vi "WLAN - niVST - RFSA - Measure.vi"(0 "IVI Refnum in":refnum<k15>="RIO0", 1 "Channel Bandwidth(Hz)":dbl=20000000.0, 2 "Path Loss dB":dbl=0.1, 3 "#Avg":i32=1, 6 "Power Level(dBm)":dbl=-10.0, 7 "Spectrum Meas Ref":T9, 8 "NIStandard":T1=enum."80211B/G(DSSS)", 10 "Center Frequency(Hz)":dbl=5190000000.0, 11 "IQ Measurement Ref":T9) -> (13 "Mod Result":T2={"EVM"=-53.23630011850784, "RMS POWER"=-20.854257366141734, "FREQ ERR PPm"=0.0031004693085368165, "Clock ERR PPm"=1.9815491854025864}, 14 "IVI Refnum out":refnum<k15>="RIO0", 15 "SMM":dbl, 16 "Margin VECTOR":dbl[](array[numeric]), 17 "Spectrum Meas Ref out":T9, 18 "IQ Measurement Ref out":T9, 19 "error out":errorcluster={"status"=TRUE, "code"=-42926, "source"="Property Node (arg 10) in niWLAN - OPPO - 80211abgnIQMeasurementsSettings.vi->WLAN - niVST - RFSA - Measure.vi->WLAN - OPPO - UUT(Tx).vi"})   [LabVIEW 2012]
uses:
  <vilib>/RF Toolkits/WLAN/analysis/controls/wlanv1 Analysis Refnum.ctl
  TV/RW/Includes/WLAN - TV - OPPO - RW - INC - TV_IQComposite_11N.ctl
  TV/RW/Includes/WLAN - TV - RW - INC - TV_OFDM Demod.ctl
  TV/RW/Includes/WLAN - TV - OPPO - RW - INC - TV_IQComposite_11B.ctl
  TV/RW/Includes/WLAN - TV - RW - INC - TV_DSSS Demod.ctl
  TV/RW/Includes/WLAN - TV - OPPO - RW - INC - TV_IQComposite_11A.ctl
  TV/RW/Includes/WLAN - TV - OPPO - RW - INC - TV_IQComposite_11AC.ctl
  TV/RW/Includes/WLAN - TV - RW - INC - Tx_IQModResult.ctl
  TV/RW/Includes/WLAN - NIStandardDefine.ctl
panel:
  in  "TV_IQComposite_11AC":T3={"Standard"=4, "OFDM Advanced Controls"={"OFDM Auto Compute Acquisition Length Enabled"=1, "OFDM Maximum Symbols Used"=16, "OFDM Time Tracking Enabled"=0, "OFDM Channel Tracking Enabled"=0, "OFDM Amplitude Tracking Enabled"=1, "OFDM CFO Estimation Method"=1, "OFDM Phase Tracking Method"=0, "OFDM Header Detection Enabled"=1, "OFDM MAC FCS Check Enabled"=0, "#Avg"=10, "#Iterations"=10}, "Measurement Enabled"=TRUE, "#Packets"=0, "Center Frequency(Hz)"=0.0, "Guard Interval (s)"=0.0, "FEC Coding Type"=0, "Generation Parameters"={"Channel BW(Hz)"=20000000.0, "MCS Index"=0, "OFDM Payload Length (bytes)"=4024, "Idle Interval(S)"=0.0, "N_SS"=0}, "Power Level(dBm)"=0.0} {"Generation Parameters"."Channel BW(Hz)" items=["5M"=5000000.0, "10M"=10000000.0, "20M"=20000000.0, "40M"=40000000.0, "80M"=80000000.0, "160M"=160000000.0]; "FEC Coding Type" items=["BCC", "LDPC"]; "Center Frequency(Hz)" format="%#_6p"; "OFDM Advanced Controls"."OFDM Phase Tracking Method" items=["Standard", "Instantaneous", "None", "Standard with Cubic Spline Fit"]; "OFDM Advanced Controls"."OFDM CFO Estimation Method" items=["Preamble Only", "Preamble and Data"]; "OFDM Advanced Controls"."OFDM Channel Tracking Enabled" items=["False", "True"]; "OFDM Advanced Controls"."OFDM Amplitude Tracking Enabled" items=["False", "True"]; "OFDM Advanced Controls"."OFDM Time Tracking Enabled" items=["True"=1, "False"=0]; "OFDM Advanced Controls"."OFDM Auto Compute Acquisition Length Enabled" items=["False", "True"]; "OFDM Advanced Controls"."OFDM MAC FCS Check Enabled" items=["False", "True"]; "OFDM Advanced Controls"."OFDM Header Detection Enabled" items=["False", "True"]; "Standard" items=["80211A/G/J/P OFDM", "80211B/G DSSS", "80211G DSSSOFDM", "80211N MIMOOFDM", "80211AC MIMOOFDM"]}
  in  "IQComp_11AG OFDM":T5={"Standard"=0, "OFDM Advanced Controls"={"OFDM Auto Compute Acquisition Length Enabled"=0, "OFDM Maximum Symbols Used"=16, "OFDM Time Tracking Enabled"=0, "OFDM Channel Tracking Enabled"=0, "OFDM Amplitude Tracking Enabled"=1, "OFDM CFO Estimation Method"=1, "OFDM Phase Tracking Method"=0, "OFDM Header Detection Enabled"=1, "OFDM MAC FCS Check Enabled"=0, "#Avg"=0, "#Iterations"=10}, "Measurement  Enabled ?"=FALSE, "#Packets"=0, "Center Frequency(Hz)"=0.0, "Power Level(dBm)"=0.0, "Payload Control"={"OFDM Data Rate (Mbps)"=0, "OFDM Payload Length (bytes)"=0, "Idle Interval (s)"=0.0}} {"Payload Control"."OFDM Data Rate (Mbps)" items=["6", "9", "12", "18", "24", "36", "48", "54"]; "Center Frequency(Hz)" format="%#_6p"; "OFDM Advanced Controls"."OFDM Phase Tracking Method" items=["Standard", "Instantaneous", "None", "Standard with Cubic Spline Fit"]; "OFDM Advanced Controls"."OFDM CFO Estimation Method" items=["Preamble Only", "Preamble and Data"]; "OFDM Advanced Controls"."OFDM Channel Tracking Enabled" items=["False", "True"]; "OFDM Advanced Controls"."OFDM Amplitude Tracking Enabled" items=["False", "True"]; "OFDM Advanced Controls"."OFDM Time Tracking Enabled" items=["True"=1, "False"=0]; "OFDM Advanced Controls"."OFDM Auto Compute Acquisition Length Enabled" items=["False", "True"]; "OFDM Advanced Controls"."OFDM MAC FCS Check Enabled" items=["False", "True"]; "OFDM Advanced Controls"."OFDM Header Detection Enabled" items=["False", "True"]; "Standard" items=["80211A/G/J/P OFDM", "80211B/G DSSS", "80211G DSSSOFDM", "80211N MIMOOFDM", "80211AC MIMOOFDM"]}
  in  "TV_IQComposite_11B":T6={"Standard"=1, "DSSS Demod Parameters"={"DSSS Auto Compute Acquisition Length Enabled"=0, "DSSS Equalization Enabled"=0, "DSSS Header Detection Enabled"=1, "DSSS MAC FCS Check Enabled"=0, "DSSS Measurement Start Location"=0, "DSSS Phase Tracking Method"=0, "DSSS Maximum Chips Used"=1000, "DSSS Reference Pulse Shaping Filter"=3, "DSSS Reference Pulse Shaping Filter Coefficient"=0.5, "# Avg"=1024, "# Iterations"=1024, "DSSS Power Ramp Enabled"=0}, "Measurement Enabled ? "=FALSE, "Power Level(dBm)"=0.0, "Center Frequency(Hz)"=0.0, "DSSS Generate Parameters"={"DSSS Data Rate (Mbps)"=0, "DSSS Payload Length (bytes)"=1024, "Idle Interval(S)"=0.0}} {"DSSS Generate Parameters"."DSSS Data Rate (Mbps)" items=["1", "2", "5.5 CCK", "5.5 PBCC", "11 CCK", "11 PBCC", "22", "33"]; "Center Frequency(Hz)" format="%#_6p"; "DSSS Demod Parameters"."DSSS Power Ramp Enabled" items=["False", "True"]; "DSSS Demod Parameters"."DSSS Auto Compute Acquisition Length Enabled" items=["False", "True"]; "DSSS Demod Parameters"."DSSS Phase Tracking Method" items=["Standard", "Instantaneous"]; "DSSS Demod Parameters"."DSSS Equalization Enabled" items=["False", "True"]; "DSSS Demod Parameters"."DSSS Reference Pulse Shaping Filter" items=["Rectangular", "Raised Cosine", "Root Raised Cosine", "Gaussian"]; "DSSS Demod Parameters"."DSSS MAC FCS Check Enabled" items=["False", "True"]; "DSSS Demod Parameters"."DSSS Header Detection Enabled" items=["False", "True"]; "Standard" items=["80211A/G/J/P OFDM", "80211B/G DSSS", "80211G DSSSOFDM", "80211N MIMOOFDM", "80211AC MIMOOFDM"]}
  in  "TV_IQComposite_11N":T8={"Standard"=3, "OFDM Advanced Controls"={"OFDM Auto Compute Acquisition Length Enabled"=0, "OFDM Maximum Symbols Used"=0, "OFDM Time Tracking Enabled"=0, "OFDM Channel Tracking Enabled"=0, "OFDM Amplitude Tracking Enabled"=1, "OFDM CFO Estimation Method"=1, "OFDM Phase Tracking Method"=0, "OFDM Header Detection Enabled"=1, "OFDM MAC FCS Check Enabled"=0, "#Avg"=10, "#Iterations"=10}, "Measurement Enabled"=FALSE, "#Packets"=0, "Guard Interval (s)"=0.0, "FEC Coding Type"=0, "80211n PLCP Frame Format"=0, "Generation Parameters"={"Channel Bandwidth(Hz)"=20000000.0, "MCS Index"=0, "OFDM Payload Length (bytes)"=4024, "Idle Interval(S)"=0.0}, "Power Level(dBm)"=0.0, "Center Frequency(Hz)"=0.0} {"Center Frequency(Hz)" format="%#_6p"; "Generation Parameters"."Channel Bandwidth(Hz)" items=["5M"=5000000.0, "10M"=10000000.0, "20M"=20000000.0, "40M"=40000000.0, "80M"=80000000.0, "160M"=160000000.0]; "80211n PLCP Frame Format" items=["Mixed Format", "Greenfield Format"]; "FEC Coding Type" items=["BCC", "LDPC"]; "OFDM Advanced Controls"."OFDM Phase Tracking Method" items=["Standard", "Instantaneous", "None", "Standard with Cubic Spline Fit"]; "OFDM Advanced Controls"."OFDM CFO Estimation Method" items=["Preamble Only", "Preamble and Data"]; "OFDM Advanced Controls"."OFDM Channel Tracking Enabled" items=["False", "True"]; "OFDM Advanced Controls"."OFDM Amplitude Tracking Enabled" items=["False", "True"]; "OFDM Advanced Controls"."OFDM Time Tracking Enabled" items=["True"=1, "False"=0]; "OFDM Advanced Controls"."OFDM Auto Compute Acquisition Length Enabled" items=["False", "True"]; "OFDM Advanced Controls"."OFDM MAC FCS Check Enabled" items=["False", "True"]; "OFDM Advanced Controls"."OFDM Header Detection Enabled" items=["False", "True"]; "Standard" items=["80211A/G/J/P OFDM", "80211B/G DSSS", "80211G DSSSOFDM", "80211N MIMOOFDM", "80211AC MIMOOFDM"]}
  in  "Data Rate (Mbps)":i32
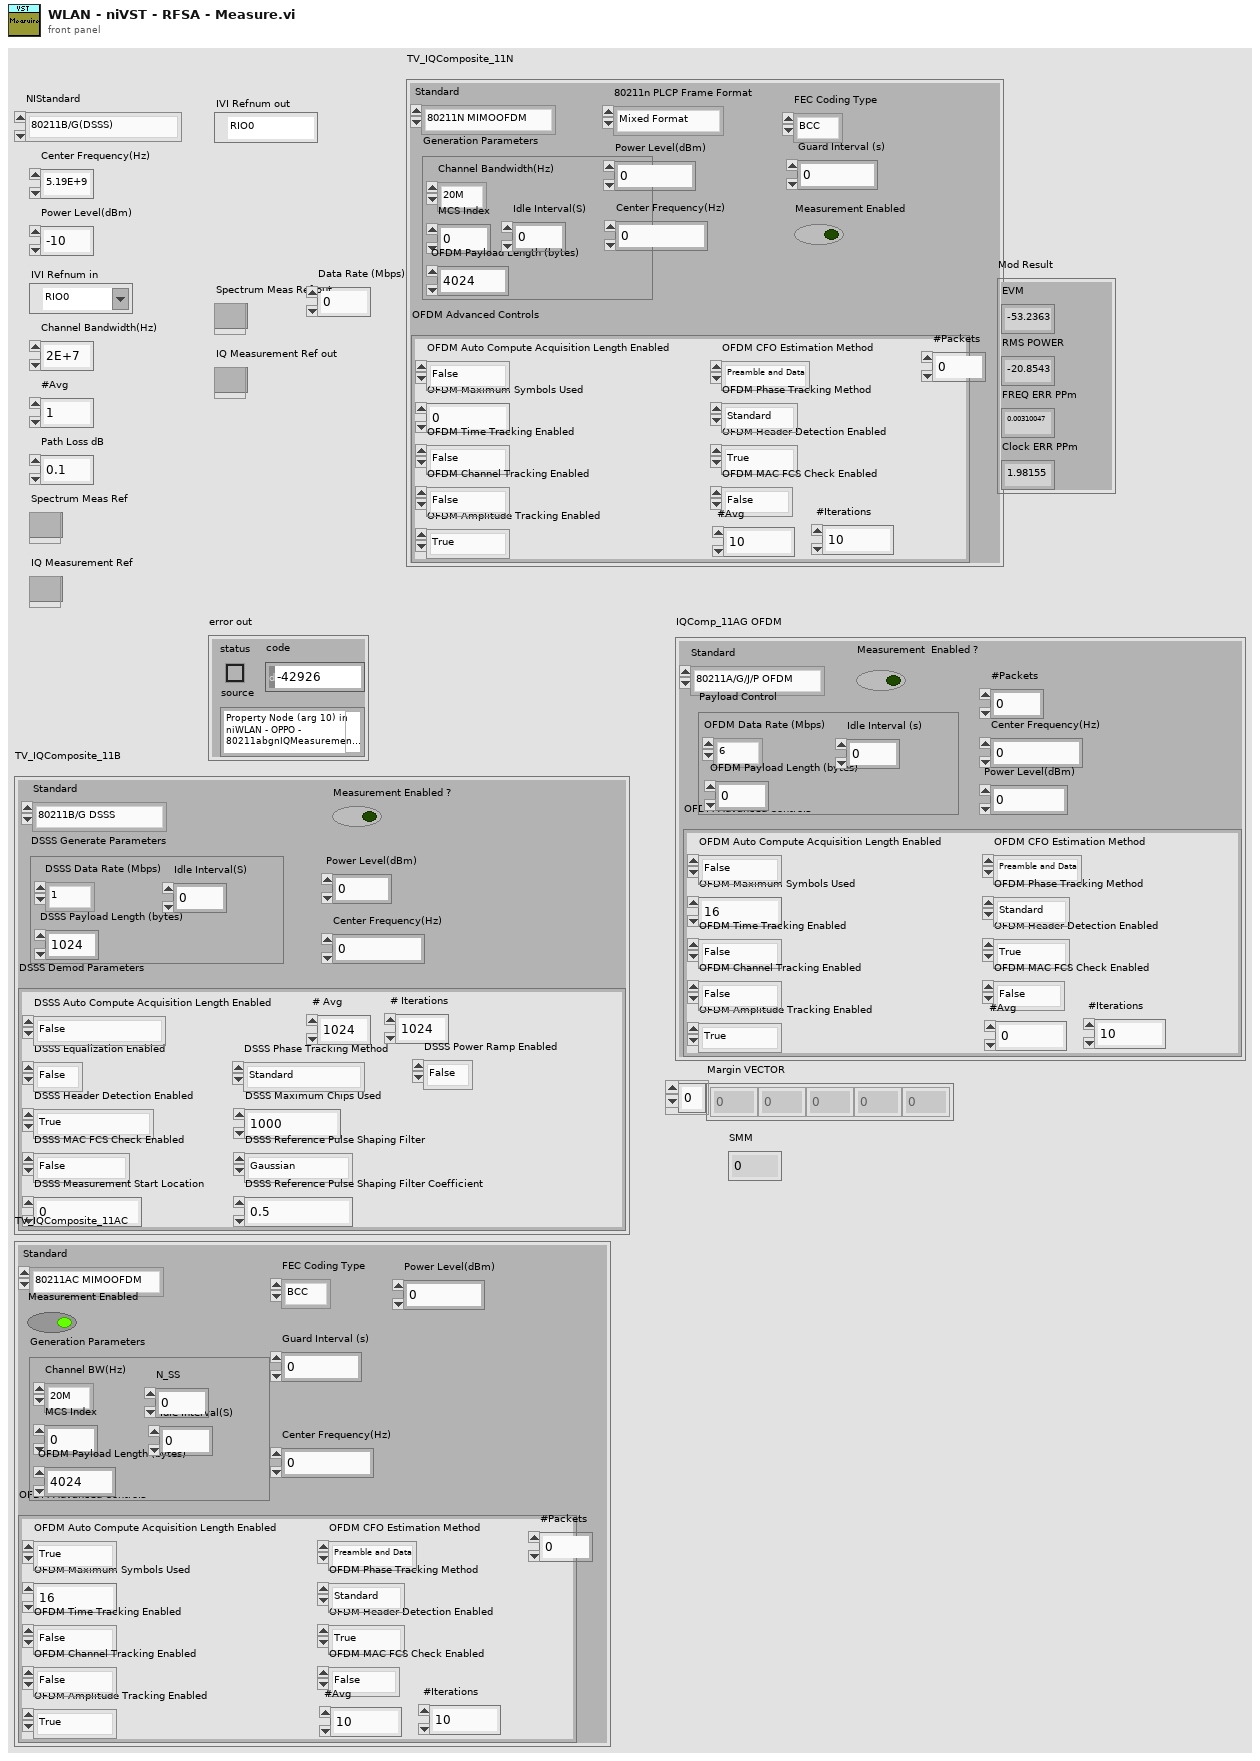
[diagram p1: front panel]
types:
  T1 = typedef "WLAN - NIStandardDefine.ctl" = enum32{"80211A/G/J/P(OFDM)", "80211B/G(DSSS)", "80211GDSSSOFDM", "80211NMIMOOFDM", "80211ACMIMOOFDM"}
  T2 = typedef "WLAN - TV - RW - INC - Tx_IQModResult.ctl" = cluster{"EVM":dbl, "RMS POWER":dbl, "FREQ ERR PPm":dbl, "Clock ERR PPm":dbl}
  T3 = typedef "WLAN - TV - OPPO - RW - INC - TV_IQComposite_11AC.ctl" = cluster{"Standard":i32, "OFDM Advanced Controls":T4, "Measurement Enabled":bool, "#Packets":i32, "Center Frequency(Hz)":dbl, "Guard Interval (s)":dbl, "FEC Coding Type":i32, "Generation Parameters":cluster{"Channel BW(Hz)":dbl, "MCS Index":i32, "OFDM Payload Length (bytes)":i32, "Idle Interval(S)":dbl, "N_SS":i32}, "Power Level(dBm)":dbl}
  T4 = typedef "WLAN - TV - RW - INC - TV_OFDM Demod.ctl" = cluster{"OFDM Auto Compute Acquisition Length Enabled":i32, "OFDM Maximum Symbols Used":i32, "OFDM Time Tracking Enabled":i32, "OFDM Channel Tracking Enabled":i32, "OFDM Amplitude Tracking Enabled":i32, "OFDM CFO Estimation Method":i32, "OFDM Phase Tracking Method":i32, "OFDM Header Detection Enabled":i32, "OFDM MAC FCS Check Enabled":i32, "#Avg":i32, "#Iterations":i32}
  T5 = typedef "WLAN - TV - OPPO - RW - INC - TV_IQComposite_11A.ctl" = cluster{"Standard":i32, "OFDM Advanced Controls":T4, "Measurement  Enabled ?":bool, "#Packets":i32, "Center Frequency(Hz)":dbl, "Power Level(dBm)":dbl, "Payload Control":cluster{"OFDM Data Rate (Mbps)":i32, "OFDM Payload Length (bytes)":i32, "Idle Interval (s)":dbl}}
  T6 = typedef "WLAN - TV - OPPO - RW - INC - TV_IQComposite_11B.ctl" = cluster{"Standard":i32, "DSSS Demod Parameters":T7, "Measurement Enabled ? ":bool, "Power Level(dBm)":dbl, "Center Frequency(Hz)":dbl, "DSSS Generate Parameters":cluster{"DSSS Data Rate (Mbps)":i32, "DSSS Payload Length (bytes)":i32, "Idle Interval(S)":dbl}}
  T7 = typedef "WLAN - TV - RW - INC - TV_DSSS Demod.ctl" = cluster{"DSSS Auto Compute Acquisition Length Enabled":i32, "DSSS Equalization Enabled":i32, "DSSS Header Detection Enabled":i32, "DSSS MAC FCS Check Enabled":i32, "DSSS Measurement Start Location":i32, "DSSS Phase Tracking Method":i32, "DSSS Maximum Chips Used":i32, "DSSS Reference Pulse Shaping Filter":i32, "DSSS Reference Pulse Shaping Filter Coefficient":dbl, "# Avg":i32, "# Iterations":i32, "DSSS Power Ramp Enabled":i32}
  T8 = typedef "WLAN - TV - OPPO - RW - INC - TV_IQComposite_11N.ctl" = cluster{"Standard":i32, "OFDM Advanced Controls":T4, "Measurement Enabled":bool, "#Packets":i32, "Guard Interval (s)":dbl, "FEC Coding Type":i32, "80211n PLCP Frame Format":i32, "Generation Parameters":cluster{"Channel Bandwidth(Hz)":dbl, "MCS Index":i32, "OFDM Payload Length (bytes)":i32, "Idle Interval(S)":dbl}, "Power Level(dBm)":dbl, "Center Frequency(Hz)":dbl}
  T9 = typedef "wlanv1 Analysis Refnum.ctl" = refnum<k20>
  T10 = cluster{"Path Loss":dbl, "Path Loss Manual ?":bool}
  T11 = enum16{"Demod Measurement", "Spectrum Measurement"}
  T12 = typedef "WLAN - TV - RW - INC - Tx_Measurement_Cluster.ctl" = cluster{"OFDM Advanced Controls(11ag)":T4, "DSSS Demod Parameters":T7, "OFDM Advanced Controls (11n)":T4, "OFDM Advanced Controls(11ac)":cluster{"OFDM Auto Compute Acquisition Length Enabled":i32, "OFDM Maximum Symbols Used":i32, "OFDM Time Tracking Enabled":i32, "OFDM Channel Tracking Enabled":i32, "OFDM Amplitude Tracking Enabled":i32, "OFDM CFO Estimation Method":i32, "OFDM Phase Tracking Method":i32, "OFDM Header Detection Enabled":i32, "OFDM MAC FCS Check Enabled":i32, "#Avg":i32, "#Iterations":i32}}
  T13 = typedef "WLAN - TV - RW - INC - TV_DataType_Cluster.ctl" = cluster{"Standard":i32, "Channel Frequency(Hz)":dbl, "Power Level(dBm)":dbl, "Channel Bandwidth (Hz)":dbl, "Idle Interval(s)":dbl, "OFDM Data Rate (Mbps)":i32, "OFDM Payload Length (bytes)":i32, "Number of Packets":i32, "MCS Index":i32, "Guard Interval (s)":dbl, "80211n PLCP Frame Format":i32, "FEC Coding Type":i32, "DSSS Data Rate (Mbps)":i32, "DSSS Payload Length (bytes)":i32, "N_SS":i32}
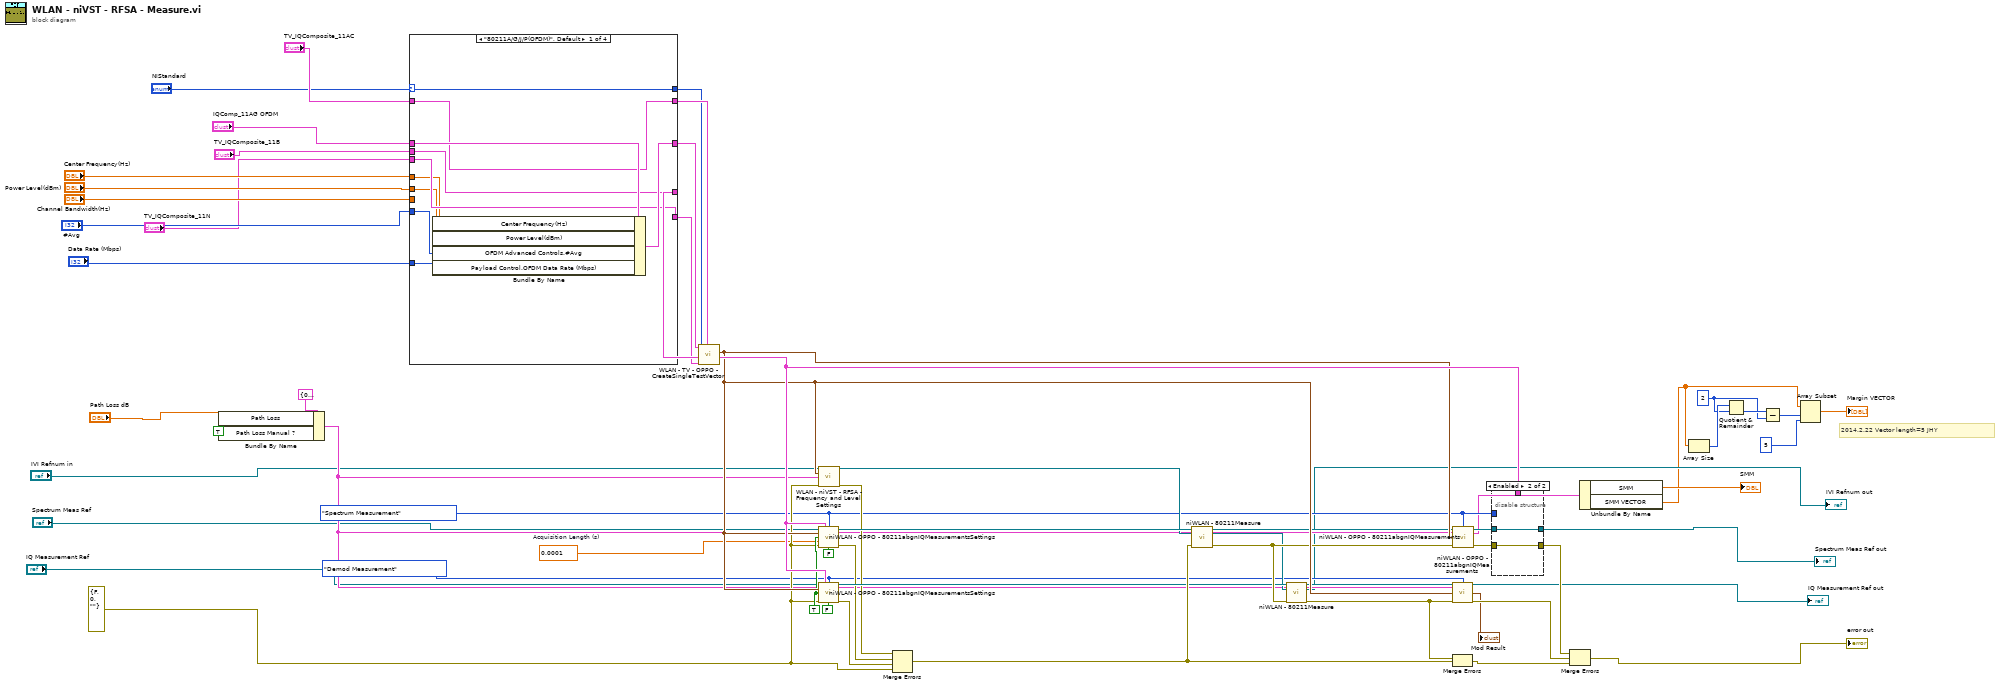
[diagram p0: block diagram]
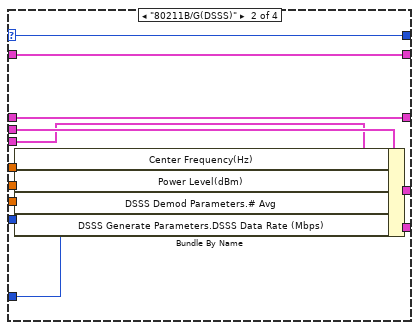
[diagram p2: hidden frame]
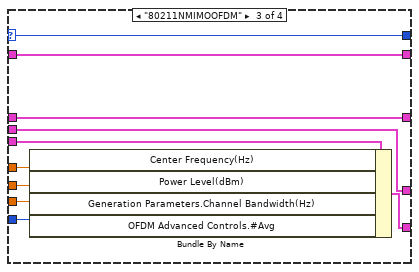
[diagram p3: hidden frame]
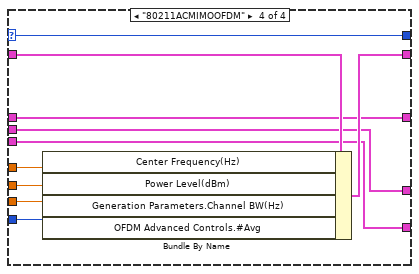
[diagram p4: hidden frame]
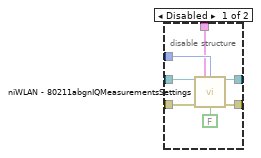
[diagram p5: hidden frame]
diagram:
  w8 = 2 ("y")
  w28 = errorcluster {"status"=FALSE, "code"=0, "source"=""} ("error in (no error)")
  w15 = 0.0001  # Acquisition Length (s)
  w48 = TRUE ("Set TV ?")
  w23 = T11."Spectrum Measurement" ("Measurement Type")
  w24 = T11."Demod Measurement" ("Measurement Type")
  # "2014.2.22 Vector length=5 JHY"
  n1 = Bundle By Name(cluster=T10 {"Path Loss"=0.0, "Path Loss Manual ?"=FALSE} ("PL"), "Path Loss"="Path Loss dB", "Path Loss Manual ?"=TRUE) -> (w26:T10)
  n2 = case shown="\"80211A/G/J/P(OFDM)\", Default" "NIStandard" {
    selector: "NIStandard" -> [w67 w77 w87 w93]
    tunnel: "TV_IQComposite_11AC" -> [w71 w79 w90 w102]
    tunnel: [w71 w79 w90 w101] -> w52
    tunnel: "IQComp_11AG OFDM" -> [w72 w80 w89 w100]
    tunnel: "TV_IQComposite_11B" -> [w69 w82 w88 w99]
    tunnel: "TV_IQComposite_11N" -> [w68 w78 w92 w98]
    tunnel: [w68 w78 w91 w98] -> w56
    tunnel: [w70 w80 w89 w100] -> w57
    tunnel: [w69 w81 w88 w99] -> w58
    tunnel: [w67 w77 w87 w93] -> w2
    tunnel: "Center Frequency(Hz)" -> [w66 w76 w86 w97]
    tunnel: "Power Level(dBm)" -> [w65 w75 w85 w96]
    tunnel: "Channel Bandwidth(Hz)" -> [_ _ w84 w95]
    tunnel: "#Avg" -> [w64 w74 w83 w94]
    tunnel: "Data Rate (Mbps)" -> [w63 w73 _ _]
    frame "80211A/G/J/P(OFDM)", Default {
      n3 = Bundle By Name(cluster=w72, "Center Frequency(Hz)"=w66, "Power Level(dBm)"=w65, "OFDM Advanced Controls.#Avg"=w64, "Payload Control.OFDM Data Rate (Mbps)"=w63) -> (w70:T5)
    }
    frame "80211B/G(DSSS)" {
      n4 = Bundle By Name(cluster=w82, "Center Frequency(Hz)"=w76, "Power Level(dBm)"=w75, "DSSS Demod Parameters.# Avg"=w74, "DSSS Generate Parameters.DSSS Data Rate (Mbps)"=w73) -> (w81:T6)
    }
    frame "80211NMIMOOFDM" {
      n5 = Bundle By Name(cluster=w92, "Center Frequency(Hz)"=w86, "Power Level(dBm)"=w85, "Generation Parameters.Channel Bandwidth(Hz)"=w84, "OFDM Advanced Controls.#Avg"=w83) -> (w91:T8)
    }
    frame "80211ACMIMOOFDM" {
      n6 = Bundle By Name(cluster=w102, "Center Frequency(Hz)"=w97, "Power Level(dBm)"=w96, "Generation Parameters.Channel BW(Hz)"=w95, "OFDM Advanced Controls.#Avg"=w94) -> (w101:T3)
    }
  }
  n7 = call "WLAN - TV - OPPO - CreateSingleTestVector.vi"("TV_IQComposite_11AC"=w52, "TV_IQComposite_11N"=w56, "TV_IQComposite_11B"=w58, "Standard"=w2, "IQComp_11AG OFDM"=w57) -> ("WLAN Measurement Settings"=w50:T12, "Tv Element"=w49:T13)  [unwired: 5 in]
  n8 = call "niWLAN - OPPO - 80211abgnIQMeasurementsSettings.vi"("niwlan analysis session"="Spectrum Meas Ref", "WLAN Measurement Settings"=w50, "Measurement Type"=w23, "TV Parameters(DataType)"=w49, "Set TV ?"=w48, "Acquisition Length (s)"=w15, "error in"=w28, "Cal Routine ?"=FALSE) -> ("niWLAN session"=w33:T9, "error out"=w34:errorcluster)  [unwired: 6 in]
  n9 = call "niWLAN - OPPO - 80211abgnIQMeasurementsSettings.vi"("niwlan analysis session"="IQ Measurement Ref", "WLAN Measurement Settings"=w50, "Measurement Type"=w24, "TV Parameters(DataType)"=w49, "Set TV ?"=w48, "error in"=w28, "Cal Routine ?"=FALSE) -> ("niWLAN session"=w37:T9, "error out"=w41:errorcluster)  [unwired: 7 in]
  n10 = call "WLAN - niVST - RFSA - Frequency and Level Settings.vi"("instrument handle"="IVI Refnum in", "TV Parameters(DataType)"=w49, "PL"=w26, "error in"=w28) -> ("instrument handle"=w30:refnum<k15>, "error out"=w29:errorcluster)  [unwired: 10 in]
  n11 = Merge Errors(w29, w34, w41, w28) -> (w47:errorcluster)
  n12 = call "niWLAN - 80211Measure.vi"("niwlan analysis session"=w33, "instrument handle"=w30, "error in"=w47) -> ("niwlan analysis session out"=w43:T9, "instrument handle out"=w36:refnum<k15>, "error out"=w44:errorcluster)  [unwired: 10 in]
  n13 = call "niWLAN - 80211Measure.vi"("niwlan analysis session"=w37, "instrument handle"=w36, "error in"=w44) -> ("niwlan analysis session out"=w38:T9, "instrument handle out"=→"IVI Refnum out":refnum<k15>, "error out"=w45:errorcluster)  [unwired: 10 in]
  n14 = call "niWLAN - OPPO - 80211abgnIQMeasurements.vi"("niwlan analysis session"=w38, "Measurement Type"=w24, "PL"=w26, "TV Parameters(DataType)"=w49, "error out"=w45) -> ("niWLAN session"=→"IQ Measurement Ref out":T9, "Mod Result"=→"Mod Result":T2, "error out"=w42:errorcluster)  [unwired: 7 in, 1 out]
  n15 = Merge Errors(w45, w47) -> (w46:errorcluster)
  n16 = call "niWLAN - OPPO - 80211abgnIQMeasurements.vi"("niwlan analysis session"=w43, "Measurement Type"=w23, "PL"=w26, "TV Parameters(DataType)"=w49, "error out"=w44) -> ("niWLAN session"=w31:T9, "Spectrum Result"=w12:cluster{"SMM":dbl, "SMM VECTOR":dbl[]}, "error out"=w32:errorcluster)  [unwired: 7 in, 1 out]
  n17 = disable-structure shown="Enabled" {
    disable-tunnel: [w109 w110] -> w19
    disable-tunnel: w23 -> [w108 _]
    disable-tunnel: w50 -> [w107 _]
    disable-tunnel: w31 -> [w106 w110]
    disable-tunnel: w32 -> [w105 w111]
    disable-tunnel: [w104 w111] -> w35
    frame Disabled {
      n18 = call "niWLAN - 80211abgnIQMeasurementsSettings.vi"("niwlan analysis session"=w106, "WLAN Measurement Settings"=w107, "Measurement Type"=w108, "error in"=w105, "Cal Routine ?"=FALSE) -> ("niWLAN session"=w109:T9, "error out"=w104:errorcluster)  [unwired: 9 in]
    }
    frame Enabled {
    }
  }
  "Spectrum Meas Ref out" <- w19
  n19 = Merge Errors(w35, w42, w46) -> (→"error out":errorcluster)
  n20 = Unbundle By Name(w12) -> ("SMM"=→"SMM":dbl, "SMM VECTOR"=w5:dbl[])
  n21 = Array Size(array=w5) -> (size(s)=w10:i32)
  n22 = Quotient & Remainder(x=w10, y=w8) -> (floor(x/y)=w9:i32)  [unwired: 1 out]
  n23 = Subtract(x=w9, y=w8) -> (x-y=w7:i32)
  n24 = Array Subset(array=w5, index=w7, length=5 ("y")) -> (→"Margin VECTOR":dbl[])
